vi "DACQH.vi"(6 "writeEqualsRead?":bool, 8 "Readback":u32) -> (0 "DACQuWriteTimeout":bool)   [LabVIEW 2014]
uses:
  <vilib>/rvi/Emulation/niFpgaSctlEmulationGetInTimedLoop.vi
  <vilib>/rvi/interface/RandomDataEmulation/niFpgaRandomDataHandleErrors.vi
  queueHandlerGlobals.vi
  <vilib>/rvi/Emulation/niFpgaProcessEmulError.vi
  <vilib>/rvi/DataTransferAndStorage/Container/XNode/niFpgaContainer.xnode
  <vilib>/rvi/interface/RandomDataEmulation/nirviRandomDataFpgaReadWriteTemplate.vi
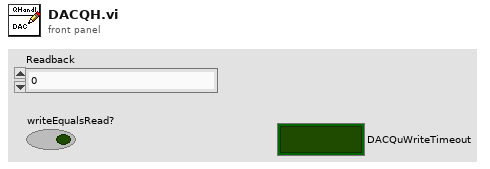
[diagram p1: front panel]
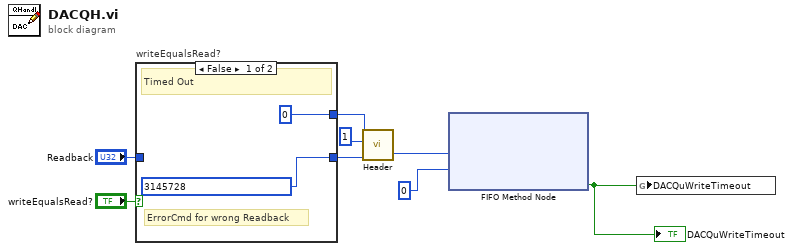
[diagram p0: block diagram]
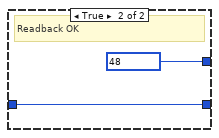
[diagram p2: hidden frame]
diagram:
  n1 = case "writeEqualsRead?" shown="False" "writeEqualsRead?" {
    tunnel: [u8 0 ("8BitHead") u8 48 ("8BitHead")] -> w8
    tunnel: "Readback" -> [_ w11]
    tunnel: [u32 3145728 ("Readback") w11] -> w4
    frame False {
      # "ErrorCmd for wrong Readback"
      # "Timed Out"
    }
    frame True {
      # "Readback OK"
    }
  }
  n2 = call "Header.vi"("23BitData"=w4, "1BitHeaderIndex"=u8 1, "8BitHead"=w8) -> ("32BitOutput"=w6:u32)  [unwired: 2 in]
  n3 = xnode ("FIFO Method Node")("Element"=w6, "Timeout"=0) -> ("Timed Out?"=w1:bool)  [unwired: 1 in, 1 out]
  "DACQuWriteTimeout" <- w1
  n4 = global write "queueHandlerGlobals.vi" "DACQuWriteTimeout"(w1) -> ()
